vi "Data Logging.vi"(2 "text":string, 3 "access (0:read/write)":enum16{"read/write", "read-only", "write-only"}(ring), 4 "error in":errorcluster, 5 "operation (0:open)":T1(ring), 6 "file":string, 7 "path":path) -> (0 "path":path, 1 "error out":errorcluster)   [LabVIEW 2019, in "SubVIs.lvlib" / "Command VI.lvlib"]
uses:
  Command VI.lvlib
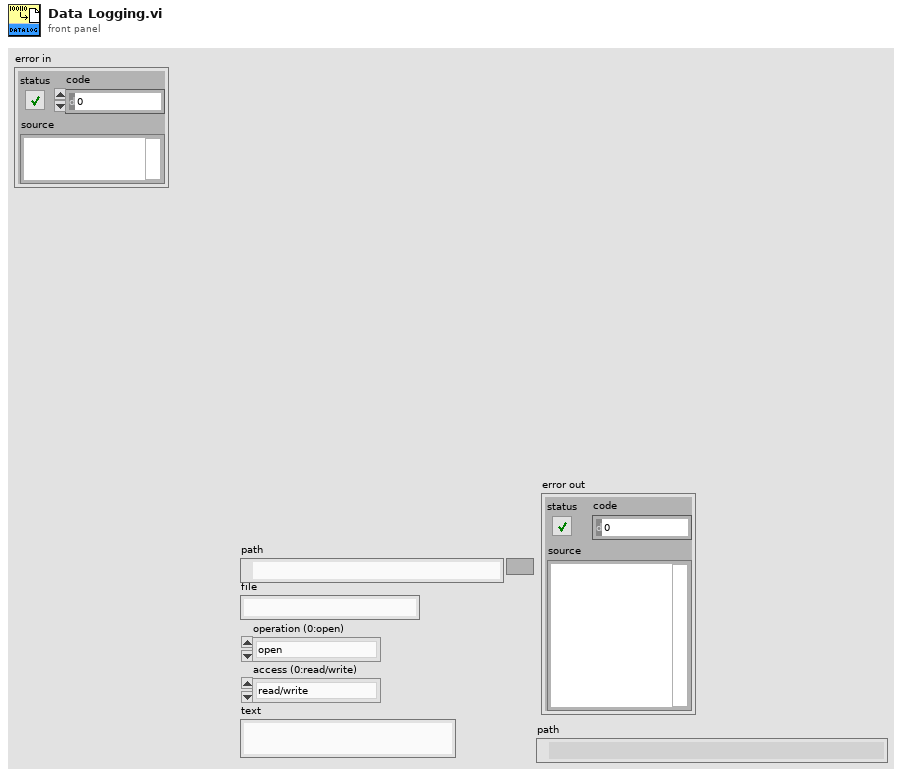
[diagram p1: front panel]
types:
  T1 = enum16{"open", "replace", "create", "open or create", "replace or create", "replace or create with confirmation"}
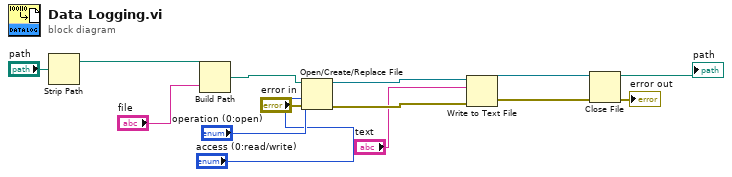
[diagram p0: block diagram]
diagram:
  n1 = Strip Path(path="path") -> (stripped path=w9:path)  [unwired: 1 out]
  n2 = Build Path(base path=w9, name or relative path="file") -> (appended path=w14:path)
  n3 = Open/Create/Replace File(file path (use dialog)=w14, error in="error in", operation (0:open)="operation (0:open)", access (0:read/write)="access (0:read/write)") -> (refnum out=w13:refnum<file>, error out=w12:errorcluster)  [unwired: 2 in, 1 out]
  n4 = Write to Text File(file (use dialog)=w13, text="text", error in=w12) -> (refnum out=w11:refnum<file>, error out=w10:errorcluster)  [unwired: 1 in, 1 out]
  n5 = Close File(refnum=w11, error in=w10) -> (path=→"path":path, error out=→"error out":errorcluster)
